vi "Destroy Test Assert Factory.vi"(8 "error in (no error)":errorcluster, 11 "Test Assert Factory in":refnum<class "Test Assert Factory.lvclass">) -> (0 "error out":errorcluster)   [LabVIEW 2013, in "Caraya.lvlib" / "Test Assert Factory.lvclass"]
uses:
  Test Assert Factory.lvclass
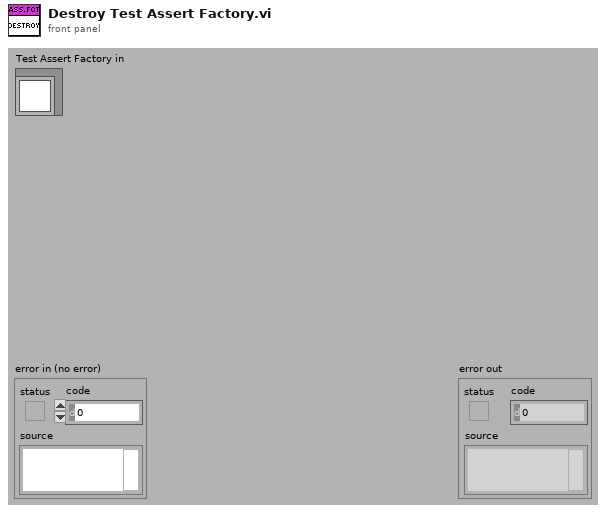
[diagram p1: front panel]
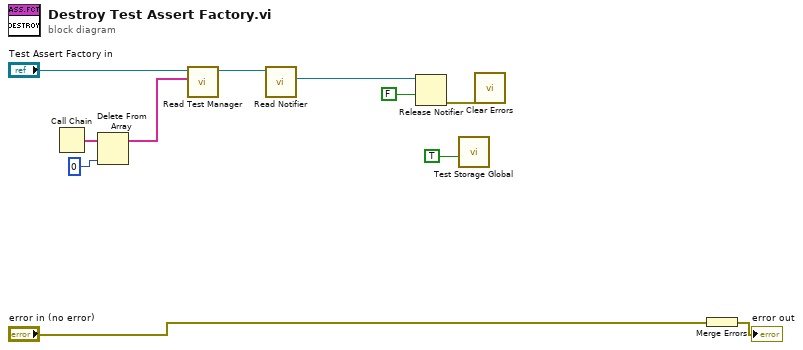
[diagram p0: block diagram]
diagram:
  n1 = Call Chain() -> (call chain=w5:string[])
  n2 = Delete From Array(array=w5, index=0) -> (array with subset deleted=w4:string[])  [unwired: 1 in, 1 out]
  n3 = call-dynamic "Read Test Manager.vi"("VI Call Chain"=w4, "Assert Factory in"="Test Assert Factory in") -> ("Assert Factory out"=w2:refnum<class "Test Assert Factory.lvclass">)  [unwired: 7 in, 2 out]
  n4 = call "Read Notifier.vi"("Test Assert Factory in"=w2) -> ("notifier"=w1:refnum<notifier>)  [unwired: 8 in, 2 out]
  n5 = Release Notifier(notifier=w1, force destroy? (F)=FALSE) -> (error out=w8:errorcluster)  [unwired: 1 in, 2 out]
  n6 = call "Test Storage Global.vi"("Clear (F)"=TRUE) -> ()  [unwired: 9 in, 2 out]
  n7 = call <vilib>:"Clear Errors.vi"("error in (no error)"=w8) -> ()  [unwired: 6 in, 1 out]
  n8 = Merge Errors("error in (no error)") -> (→"error out":errorcluster)
